vi "IScanShutter.vi"(3 "OpenNotClose":i32, 4 "Shutter #":i32=1, 5 "PRIORLib.IScanIn":refnum<k7>) -> (0 "Return":i32, 1 "error out":errorcluster, 2 "PRIORLib.IScanOut":refnum<k7>)   [LabVIEW 2011]
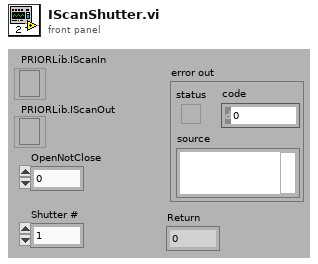
[diagram p1: front panel]
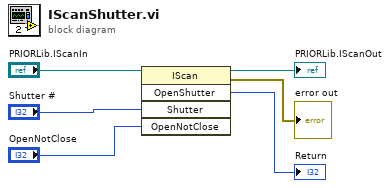
[diagram p0: block diagram]
diagram:
  n1 = invoke class="IScan" method="OpenShutter"(reference="PRIORLib.IScanIn", "Shutter"="Shutter #", "OpenNotClose"="OpenNotClose") -> (reference out=→"PRIORLib.IScanOut":refnum<k7>, error out=→"error out":errorcluster, "OpenShutter"=→"Return":i32)  [unwired: 2 in, 2 out]
